vi "hash2hex.vi"(11 "hash string":string) -> (3 "hex string":string)   [LabVIEW 2015, in "LV Interface for Amazon S3.lvlib"]
uses:
  LV Interface for Amazon S3.lvlib
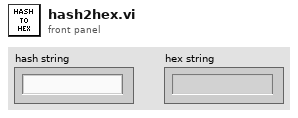
[diagram p1: front panel]
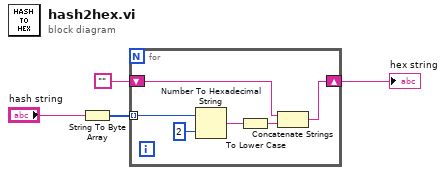
[diagram p0: block diagram]
diagram:
  n1 = String To Byte Array(string="hash string") -> (unsigned byte array=w3:u8[])
  n2 = for {
    shift-right: [w7] -> w4
    shift-left: "" -> [w8]
    tunnel: w3 -> [w10] mode=indexing
    n3 = Number To Hexadecimal String(1:i16 2 ("width (-)"), 2:w10) -> (0:w6:string)
    n4 = To Lower Case(string=w6) -> (all lower case string=w5:string)
    n5 = Concatenate Strings(w8, w5) -> (w7:string)
  }
  "hex string" <- w4
